vi "Final.vi"() -> ()   [LabVIEW 2020]
uses:
  <vilib>/MakerHub/LINX/Public/Utilities/Open Serial.vi
  <vilib>/MakerHub/LINX/LMH-LINX.lvlib
panel:
  in  "lm35 pin":u8
  in  "Relay Fan DO Channel":u8
  in  "Serial Port":refnum<visa-resource-name>="N/A"
  out "Waveform Chart moisture":dbl(graph)
  in  "PwmpinLedMoisture":u8
  in  "Analog Channe for soil moisturel":u8
  out "U1 Distance(cm)":u32
  in  "Echo 2":u8
  in  "Echo":u8
  in  "Trigger":u8
  in  "Trigger 2":u8
  out "Waveform Chart u1\n 2":dbl(graph)
  out "Pulse Width (uS) 3":u32
  out "U1 Distance(cm) 2":u32
  out "Pulse Width (uS) 2":u32
  out "Pulse Width (uS)":u32
  in  "LDR Analog pin":u8
  in  "Enable PWM Channel for  motor":u8
  in  "IN1 Motor":u8
  in  "IN2 Motor":u8
  in  "stop":bool
  # "Light sensor"
  # "Motor Controller"
  # "Smart\nGreen House Controller"
  # "Ultra Sonic Sensor"
  # "Temperature Controller"
  # "Moisture Controller"
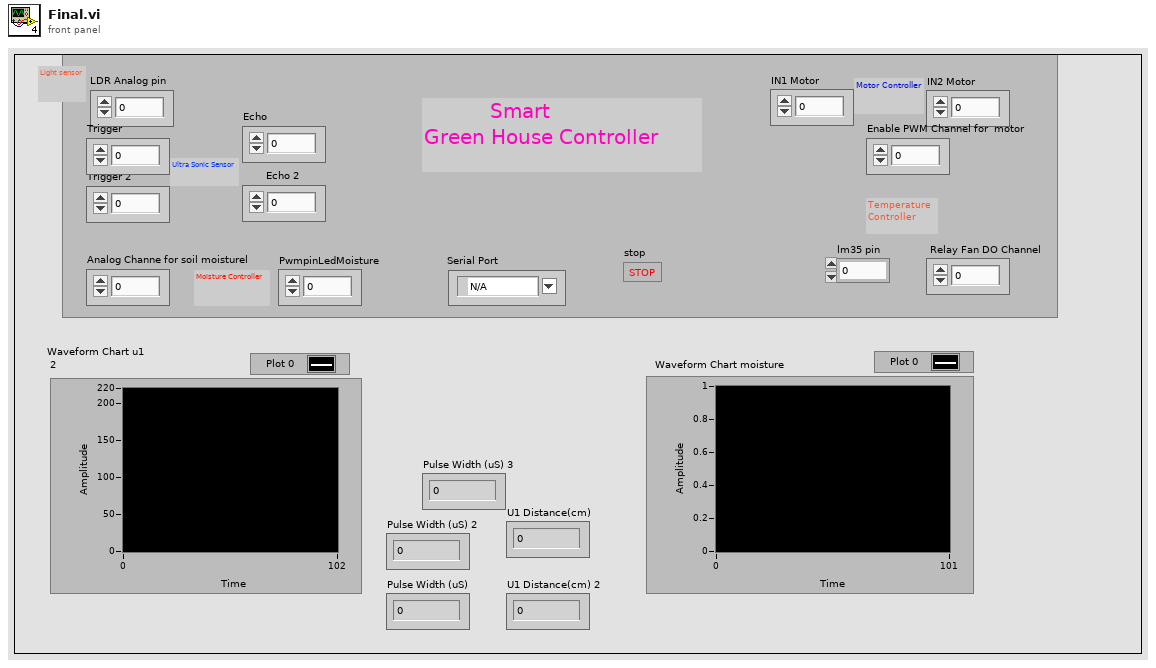
[diagram p1: front panel]
types:
  T1 = typedef "LMH-LINX.lvlib/LINX Ref.ctl" = cluster{"IO":T2, "Interface":T3, "LINX Device Config":T4}
  T2 = typedef "LMH-LINX.lvlib/Platform.ctl" = enum16{"Remote", "Local"}
  T3 = typedef "LMH-LINX.lvlib/Interface.ctl" = enum16{"Serial", "TCP"}
  T4 = typedef "LMH-LINX.lvlib/Device.lvlib/LINX Device Config.ctl" = cluster{"Interface":T3, "COM Port":refnum<visa-resource-name>, "TCP Configuration":T5, "Device Family":u8, "Device ID":u8, "Device Name":string, "TCP Ref":refnum<k5>, "Channels":T6}
  T5 = typedef "LMH-LINX.lvlib/Device.lvlib/TCP Config.ctl" = cluster{"IP Address":string, "Port":u16}
  T6 = typedef "LMH-LINX.lvlib/Channels.ctl" = cluster{"DI":u8[], "DO":u8[], "AI":u8[], "AO":u8[], "PWM":u8[], "QE":u8[], "UART":u8[], "I2C 2":u8[], "SPI":u8[], "CAN":u8[], "Servo":u8[], "AI Ref (V)":dbl, "AI Resolution (Bits)":u8, "AO Ref (V)":dbl, "AO Resolution (Bits)":u8}
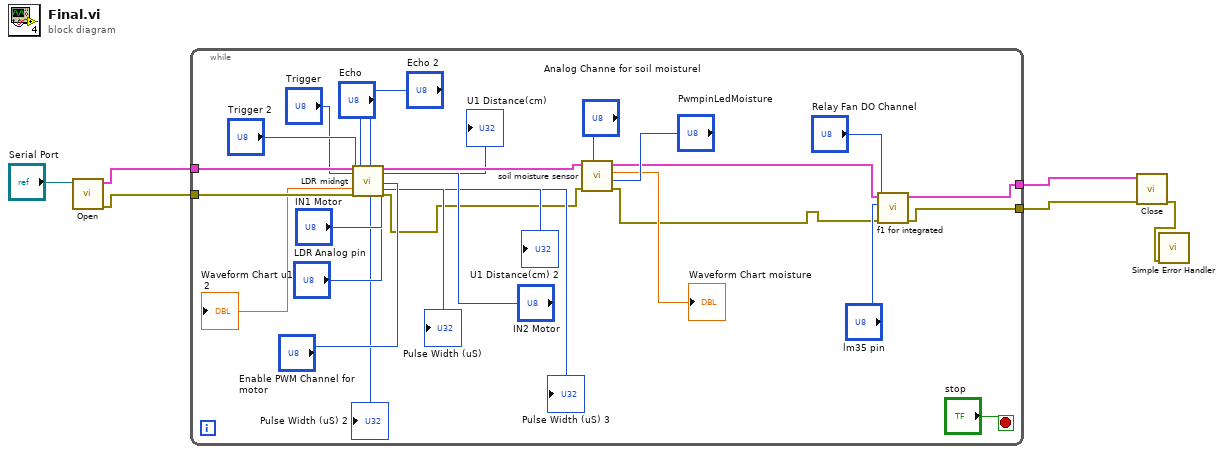
[diagram p0: block diagram]
diagram:
  n1 = call-poly <vilib>:"Open.vi"("Serial Port"="Serial Port") -> ("Error Out"=w5:errorcluster, "LINX Resource"=w6:T1)  [unwired: 8 in, 1 out]
  n2 = while {
    tunnel: w6 -> [w31]
    tunnel: w5 -> [w30]
    tunnel: [w12] -> w4
    tunnel: [w13] -> w3
    stop <- "stop" stop-if-true
    n3 = call "LDR midngt.vi"("LINX Resource"=w31, "Trigger"="Trigger", "Trigger 2"="Trigger 2", "Error Out"=w30, "Echo"="Echo", "Echo 2"="Echo 2", "IN2 Motor"="IN2 Motor", "IN1 Motor"="IN1 Motor", "Enable PWM Channel for  motor"="Enable PWM Channel for  motor", "LDR Analog pin"="LDR Analog pin") -> ("Waveform Chart u1\n 2"=→"Waveform Chart u1\n 2":dbl, "Pulse Width (uS)"=→"Pulse Width (uS)" →"Pulse Width (uS) 2":u32, "Pulse Width (uS) 2"=→"Pulse Width (uS) 3":u32, "U1 Distance(cm)"=→"U1 Distance(cm)":u32, "U1 Distance(cm) 2"=→"U1 Distance(cm) 2":u32, "LINX Resource 2"=w32:T1, "Error Out 2"=w8:errorcluster)  [unwired: 3 in]
    n4 = call "soil moisture sensor.vi"("Error Out"=w8, "PwmpinLedMoisture"="PwmpinLedMoisture", "Analog Channe for soil moisturel"="Analog Channe for soil moisturel", "LINX Resource"=w32) -> ("Error Out 2"=w7:errorcluster, "Waveform Chart moisture"=→"Waveform Chart moisture":dbl, "LINX Resource 2"=w11:T1)  [unwired: 5 in]
    n5 = call "f1 for integrated.vi"("Error Out"=w7, "Relay Fan DO Channel"="Relay Fan DO Channel", "lm35 pin"="lm35 pin", "LINX Resource"=w11) -> ("Error Out 2"=w13:errorcluster, "LINX Resource 2"=w12:T1)  [unwired: 6 in]
  }
  n6 = call <vilib>:"Close.vi"("Error In"=w3, "LINX Resource"=w4) -> ("Error Out"=w1:errorcluster)  [unwired: 9 in]
  n7 = call <vilib>:"Simple Error Handler.vi"("error in (no error)"=w1) -> ()  [unwired: 4 in, 5 out]
